vi "SW_Get_Ports_IO_and_Inv_config.vi"(5 "IO parameters cluster input":T2={"IO general config."=12, "IO 1 configuration"=1, "IO 2 configuration"=1, "IO 3 configuration"=0, "IO 4 configuration"=0, "Activate ext. RS-232"=0, "IO inversion config."=0, "Sync capability"=0}) -> (0 "IO inversion config.":u16, 1 "Ports IO config (OUT is FALSE)":bool[](array[boolean]), 2 "Zones out config bin":bool[](array[boolean]), 3 "Zones out config":u32, 4 "IO status indicator 2":T1)   [LabVIEW 2018, in "Common_Resources.lvlib"]
uses:
  Common_Resources.lvlib
  SubVi's/Controls/CTL_IO_params_cluster.ctl
  Typedefs/CTL_IO_status_indicator_2.ctl
panel:
  out "Error Out":errorcluster
  in  "Error In":errorcluster
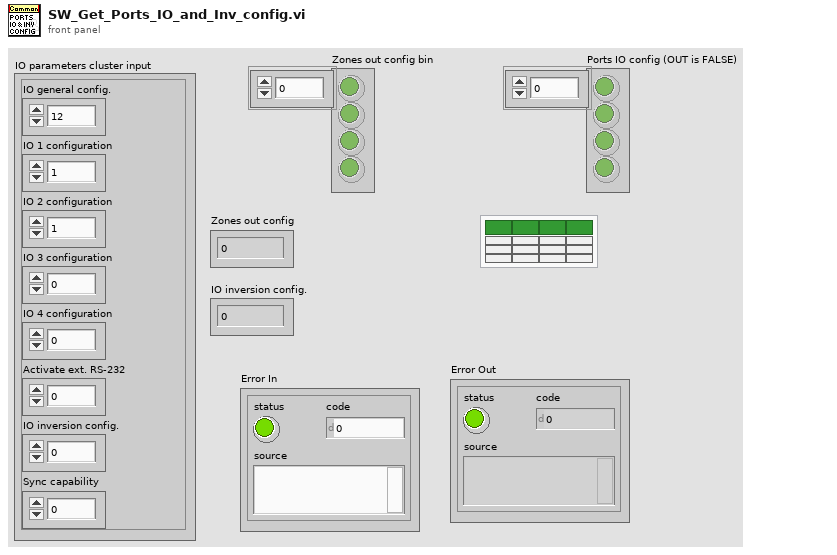
[diagram p1: front panel]
types:
  T1 = typedef "Common_Resources.lvlib/CTL_IO_status_indicator_2.ctl" = cluster{"IO1":bool, "IO2":bool, "IO3":bool, "IO4":bool, "St1":bool, "St2":bool, "St3":bool, "St4":bool, "Ext1":bool, "Ext2":bool, "Ext3":bool, "Ext4":bool, "Syn1":bool, "Syn2":bool, "Syn3":bool, "Syn4":bool}
  T2 = typedef "Common_Resources.lvlib/CTL_IO_params_cluster.ctl" = cluster{"IO general config.":u16, "IO 1 configuration":u16, "IO 2 configuration":u16, "IO 3 configuration":u16, "IO 4 configuration":u16, "Activate ext. RS-232":u16, "IO inversion config.":u16, "Sync capability":u8}
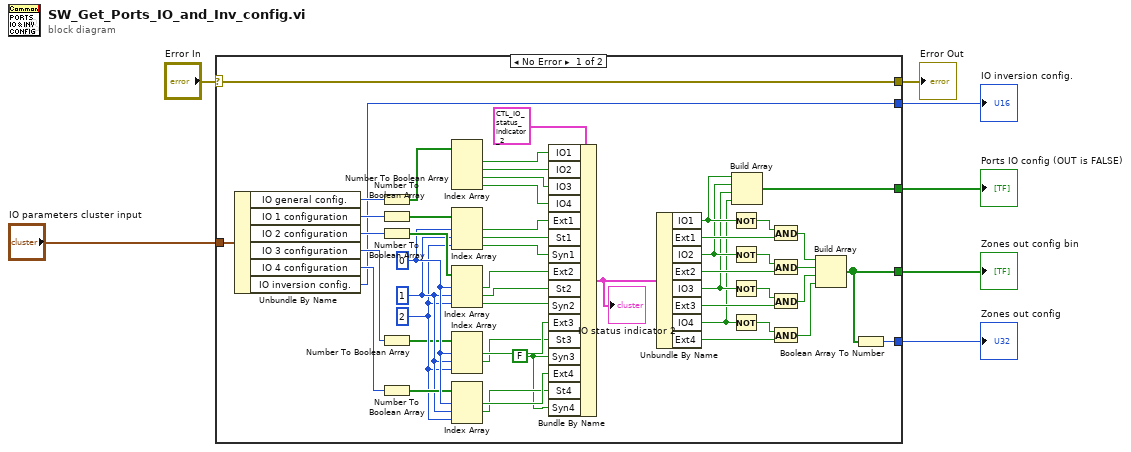
[diagram p0: block diagram]
diagram:
  n1 = case shown="No Error" "Error In" {
    selector: "Error In" -> [w31 w60]
    tunnel: "IO parameters cluster input" -> [w51 _]
    tunnel: [w34 _] -> w5
    tunnel: [w33 _] -> w4
    tunnel: [w32 _] -> w3
    tunnel: [w31 w60] -> w2
    tunnel: [w30 _] -> w1
    frame No Error {
      w8 = FALSE ("Syn3")
      w17 = 2 ("index")
      w18 = 1 ("index")
      w20 = 0 ("index")
      n2 = Unbundle By Name(w51) -> ("IO general config."=w58:u16, "IO 1 configuration"=w56:u16, "IO 2 configuration"=w54:u16, "IO 3 configuration"=w53:u16, "IO 4 configuration"=w52:u16, "IO inversion config."=w30:u16)
      n3 = Number To Boolean Array(number=w58) -> (Boolean array=w57:bool[])
      n4 = Number To Boolean Array(number=w56) -> (Boolean array=w55:bool[])
      n5 = Number To Boolean Array(number=w54) -> (Boolean array=w21:bool[])
      n6 = Number To Boolean Array(number=w53) -> (Boolean array=w16:bool[])
      n7 = Number To Boolean Array(number=w52) -> (Boolean array=w19:bool[])
      n8 = Index Array(array=w57) -> (element #1=w59:bool, element #2=w28:bool, element #3=w27:bool, element #4=w26:bool)  [unwired: 4 in]
      n9 = Index Array(array=w55, index #1=w20, index #2=w18, index #3=w17) -> (element #1=w24:bool, element #2=w23:bool, element #3=w22:bool)
      n10 = Index Array(array=w21, index #1=w20, index #2=w18, index #3=w17) -> (element #1=w15:bool, element #2=w14:bool, element #3=w13:bool)
      n11 = Index Array(array=w16, index #1=w20, index #2=w18, index #3=w17) -> (element #1=w12:bool, element #2=w11:bool)  [unwired: 1 out]
      n12 = Index Array(array=w19, index #1=w20, index #2=w18, index #3=w17) -> (element #1=w10:bool, element #2=w9:bool)  [unwired: 1 out]
      n13 = Bundle By Name(cluster=T1 {"IO1"=FALSE, "IO2"=FALSE, "IO3"=FALSE, "IO4"=FALSE, "St1"=FALSE, "St2"=FALSE, "St3"=FALSE, "St4"=FALSE, "Ext1"=FALSE, "Ext2"=FALSE, "Ext3"=FALSE, "Ext4"=FALSE, "Syn1"=FALSE, "Syn2"=FALSE, "Syn3"=FALSE, "Syn4"=FALSE} ("IO status indicator"), "IO1"=w59, "IO2"=w28, "IO3"=w27, "IO4"=w26, "Ext1"=w24, "St1"=w23, "Syn1"=w22, "Ext2"=w15, "St2"=w14, "Syn2"=w13, "Ext3"=w12, "St3"=w11, "Syn3"=w8, "Ext4"=w10, "St4"=w9, "Syn4"=w8) -> (w25:T1)
      "IO status indicator 2" <- w25
      n14 = Unbundle By Name(w25) -> ("IO1"=w38:bool, "Ext1"=w42:bool, "IO2"=w37:bool, "Ext2"=w41:bool, "IO3"=w36:bool, "Ext3"=w40:bool, "IO4"=w35:bool, "Ext4"=w39:bool)
      n15 = Not(x=w38) -> (.not. x?=w50:bool)
      n16 = Not(x=w37) -> (.not. x?=w49:bool)
      n17 = Not(x=w36) -> (.not. x?=w48:bool)
      n18 = Not(x=w35) -> (.not. x?=w47:bool)
      n19 = Build Array(w38, w37, w36, w35) -> (w32:bool[])
      n20 = And(x=w50, y=w42) -> (x .and. y?=w46:bool)
      n21 = And(x=w49, y=w41) -> (x .and. y?=w45:bool)
      n22 = And(x=w48, y=w40) -> (x .and. y?=w44:bool)
      n23 = And(x=w47, y=w39) -> (x .and. y?=w43:bool)
      n24 = Build Array(w46, w45, w44, w43) -> (w33:bool[])
      n25 = Boolean Array To Number(Boolean array=w33) -> (number=w34:u32)
    }
    frame Error {
    }
  }
  "Error Out" <- w2
  "Zones out config" <- w5
  "Zones out config bin" <- w4
  "Ports IO config (OUT is FALSE)" <- w3
  "IO inversion config." <- w1
